vi "test-filter.vi"() -> ()   [LabVIEW 2019]
uses:
  <vilib>/Rock Robotics/WPI/ThirdParty/JAS_Junk/TrajLib/LINEAR_FILTER.ctl
  <vilib>/Rock Robotics/WPI/ThirdParty/JAS_Junk/TrajLib/Trajectory_Library.lvlib
panel:
  in  "Random noise amplitude":bool
  out "time diff":u32
  out "High BW2":T1 {"Outputs" format="%13.5p"; "Inputs" format="%13.5p"; "OutputGains" format="%13.5p"; "InputGains" format="%13.5p"}
  in  "noise Offset - millliseconds":dbl format="%14.5g"
  out "Cutoff Freq":dbl format="%14.5g"
  out "High BW1":T1 {"Outputs" format="%13.5p"; "Inputs" format="%13.5p"; "OutputGains" format="%13.5p"; "InputGains" format="%13.5p"}
  out "High Pass":T1 {"Outputs" format="%13.5p"; "Inputs" format="%13.5p"; "OutputGains" format="%13.5p"; "InputGains" format="%13.5p"}
  out "mov Avg":T1 {"Outputs" format="%13.5p"; "Inputs" format="%13.5p"; "OutputGains" format="%13.5p"; "InputGains" format="%13.5p"}
  in  "MovAvgSamp":i32 format="%14.5g"
  out "BW 2":T1 {"Outputs" format="%13.5p"; "Inputs" format="%13.5p"; "OutputGains" format="%13.5p"; "InputGains" format="%13.5p"}
  out "BW 1":T1 {"Outputs" format="%13.5p"; "Inputs" format="%13.5p"; "OutputGains" format="%13.5p"; "InputGains" format="%13.5p"}
  out "Single pole":T1 {"Outputs" format="%13.5p"; "Inputs" format="%13.5p"; "OutputGains" format="%13.5p"; "InputGains" format="%13.5p"}
  in  "Noise Amplitude":dbl(slide)=1.0 scale=0.0..10.0
  in  "TimeConstant":dbl format="%14.5g"
  in  "Noise Frequency":dbl(slide)=0.2 min=0.1 max=1000.0 step=0.5 scale=0.1..1000.0 scale format="%14.5g"
  out "Waveform Chart":T2(graph)
  in  "Primary Frequency":dbl(slide)=0.2 min=0.1 max=1000.0 step=0.5 scale=0.1..10.0 scale format="%14.5g"
  in  "Amplitude":dbl(slide)=1.0 scale=0.0..10.0
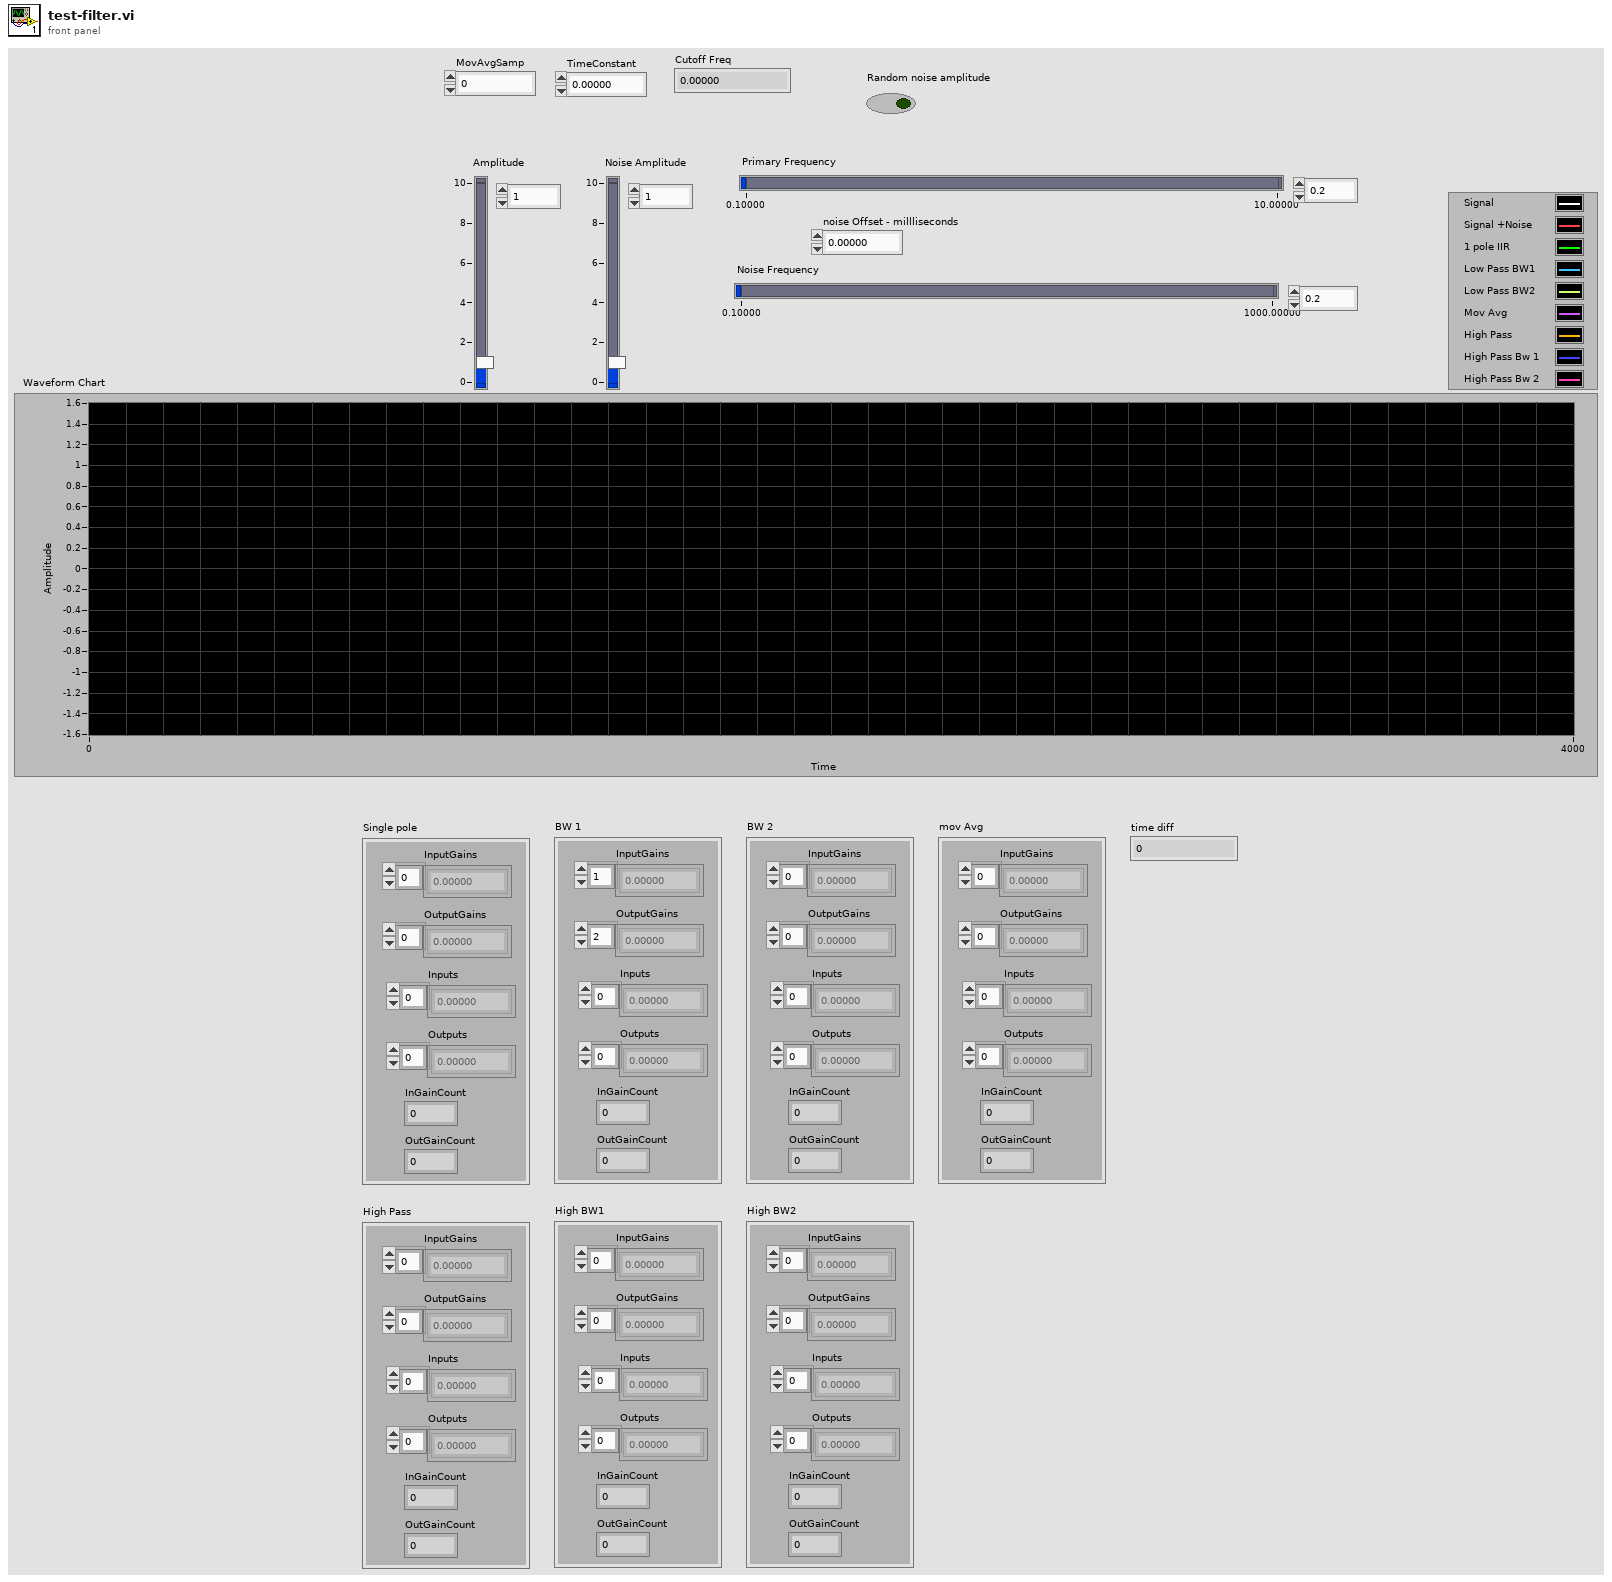
[diagram p1: front panel]
types:
  T1 = typedef "Trajectory_Library.lvlib/LINEAR_FILTER.ctl" = cluster{"InputGains":dbl[], "OutputGains":dbl[], "Inputs":dbl[], "Outputs":dbl[], "InGainCount":i32, "OutGainCount":i32}
  T2 = cluster{dbl, dbl, "Output":dbl, "Output":dbl, "Output":dbl, "Output":dbl, "Output":dbl, "Output":dbl, "Output":dbl}
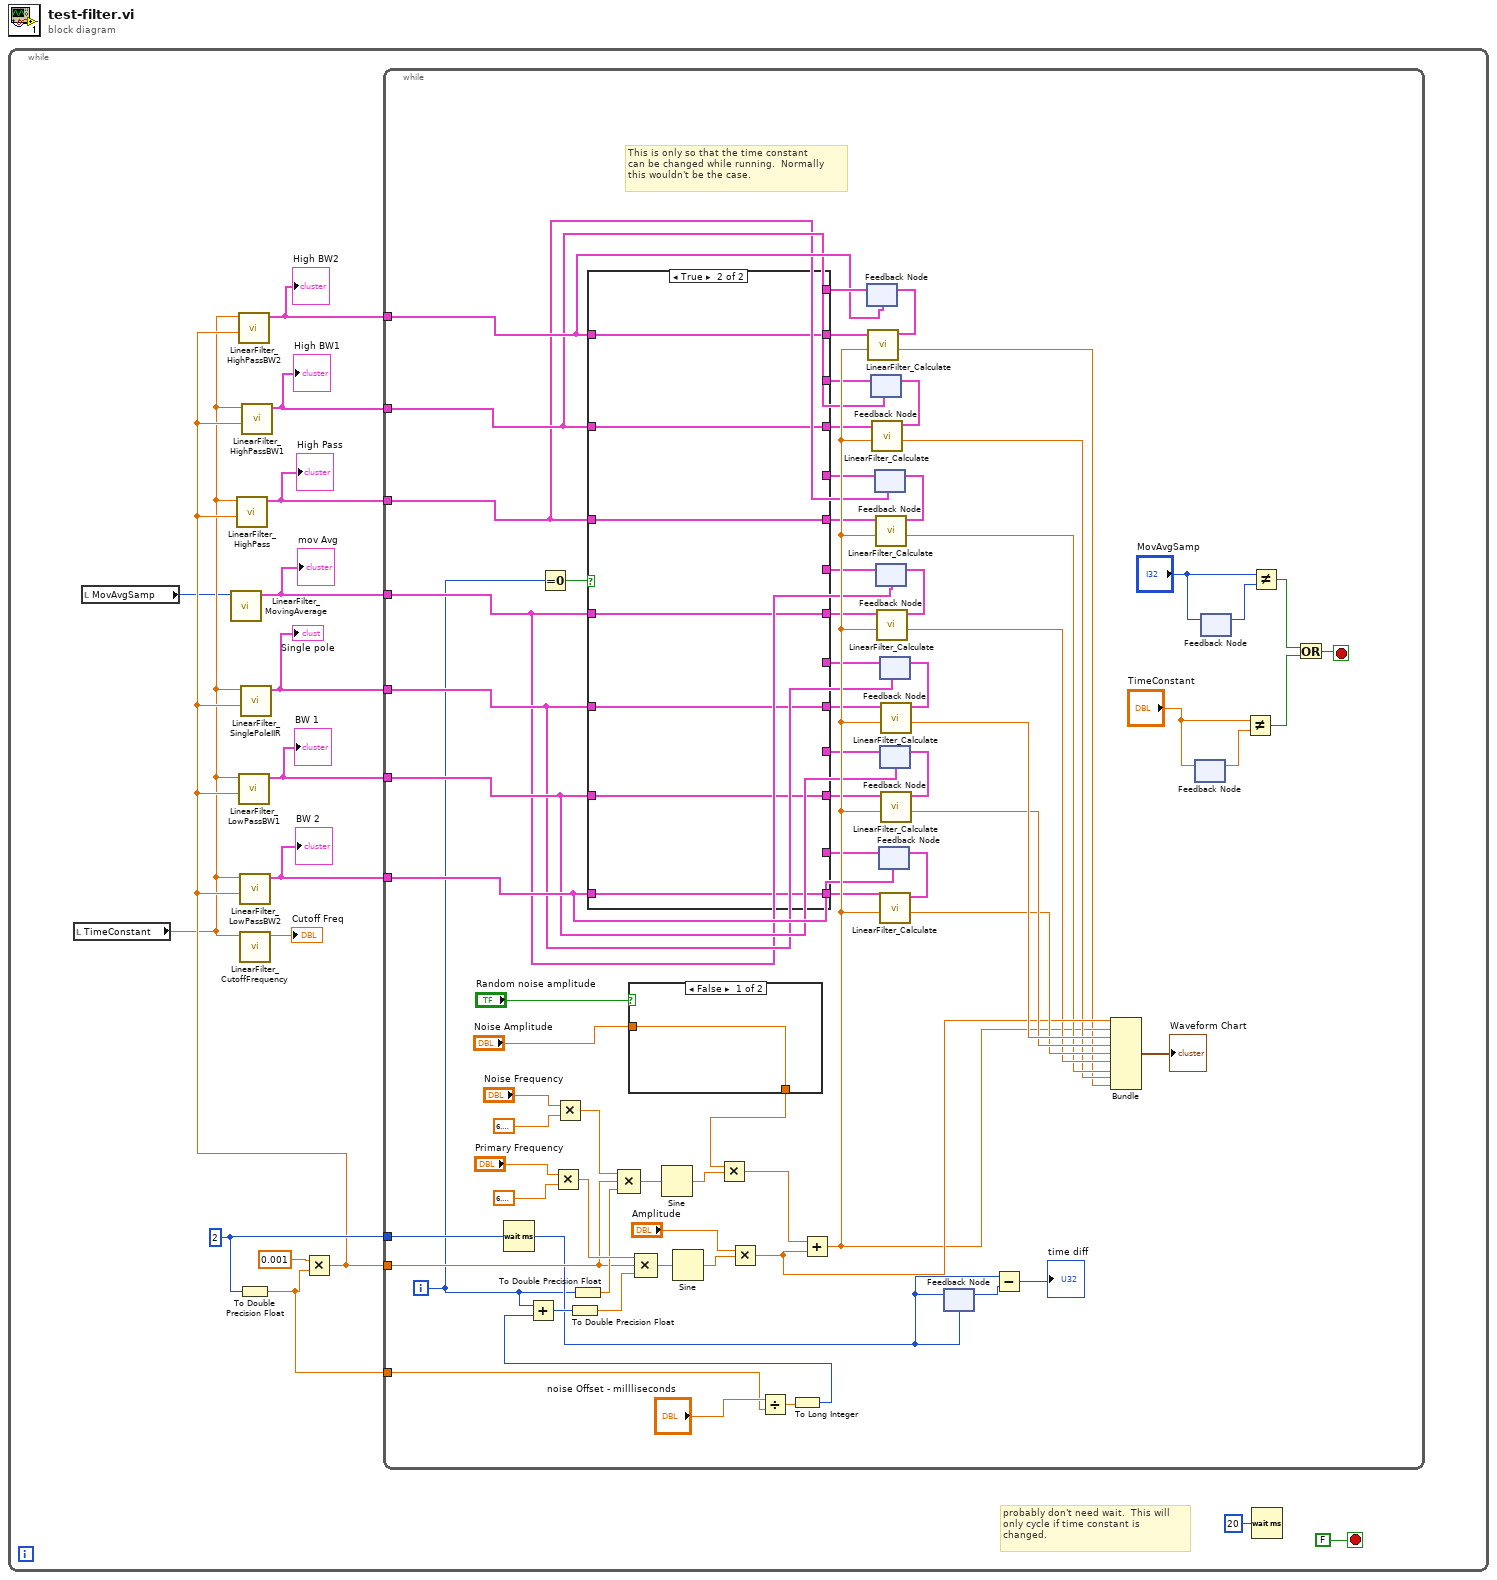
[diagram p0: block diagram]
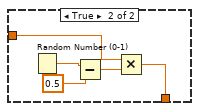
[diagram p2: hidden frame]
diagram:
  n1 = while {
    stop <- FALSE stop-if-true
    w15 = u32 2 ("milliseconds to wait")
    # "probably don't need wait.  This will \nonly cycle if time constant is\nchanged."
    n2 = local read "TimeConstant"() -> (w3:dbl)
    n3 = local read "MovAvgSamp"() -> (w2:i32)
    n4 = call <vilib>:"LinearFilter_MovingAverage.vi"("Samples"=w2) -> ("LINEAR_FILTER"=w12:T1)  [unwired: 10 in]
    "mov Avg" <- w12
    n5 = call <vilib>:"LinearFilter_CutoffFrequency.vi"("TimeConstant"=w3) -> ("Cutoff Freq"=→"Cutoff Freq":dbl)  [unwired: 10 in]
    n6 = To Double Precision Float(number=w15) -> (double precision float=w9:dbl)
    n7 = Multiply(x=0.001 ("value"), y=w9) -> (x*y=w8:dbl)
    n8 = call <vilib>:"LinearFilter_HighPass.vi"("SamplePeriod"=w8, "TimeConstant"=w3) -> ("LINEAR_FILTER"=w11:T1)  [unwired: 9 in]
    "High Pass" <- w11
    n9 = call <vilib>:"LinearFilter_HighPassBW2.vi"("SamplePeriod"=w8, "TimeConstant"=w3) -> ("LINEAR_FILTER"=w7:T1)  [unwired: 9 in]
    "High BW2" <- w7
    n10 = call <vilib>:"LinearFilter_LowPassBW1.vi"("SamplePeriod"=w8, "TimeConstant"=w3) -> ("LINEAR_FILTER"=w14:T1)  [unwired: 9 in]
    "BW 1" <- w14
    n11 = call <vilib>:"LinearFilter_LowPassBW2.vi"("SamplePeriod"=w8, "TimeConstant"=w3) -> ("LINEAR_FILTER"=w13:T1)  [unwired: 9 in]
    "BW 2" <- w13
    n12 = call <vilib>:"LinearFilter_SinglePoleIIR.vi"("SamplePeriod"=w8, "TimeConstant"=w3) -> ("LINEAR_FILTER"=w1:T1)  [unwired: 8 in, 1 out]
    "Single pole" <- w1
    n13 = call <vilib>:"LinearFilter_HighPassBW1.vi"("SamplePeriod"=w8, "TimeConstant"=w3) -> ("LINEAR_FILTER"=w10:T1)  [unwired: 9 in]
    "High BW1" <- w10
    n14 = while {
      tunnel: w15 -> [w84]
      tunnel: w8 -> [w76]
      tunnel: w14 -> [w27]
      tunnel: w13 -> [w28]
      tunnel: w12 -> [w25]
      tunnel: w11 -> [w22]
      tunnel: w10 -> [w23]
      tunnel: w9 -> [w57]
      tunnel: w7 -> [w24]
      tunnel: w1 -> [w26]
      i -> [w20]
      stop <- w45 stop-if-true
      # "This is only so that the time constant\ncan be changed while running.  Normally\nthis wouldn't be the case."
      n15 = Wait (ms)(milliseconds to wait=w84) -> (millisecond timer value=w51:u32)
      n16 = Equal To 0?(x=w20) -> (x = 0?=w21:bool)
      n17 = Multiply(x="Primary Frequency", y=6.283185307179586) -> (x*y=w78:dbl)
      n18 = Multiply(x="Noise Frequency", y=6.283185307179586) -> (x*y=w79:dbl)
      n19 = To Double Precision Float(number=w20) -> (double precision float=w77:dbl)
      n20 = Compound Arithmetic op=MULTIPLY(w79, w76, w77) -> (w81:dbl)
      n21 = case shown="False" "Random noise amplitude" {
        tunnel: "Noise Amplitude" -> [w91 w93]
        tunnel: [w91 w92] -> w17
        frame False {
        }
        frame True {
          n22 = Random Number (0-1)() -> (number: 0 to 1=w96:dbl)
          n23 = Subtract(x=w96, y=0.5) -> (x-y=w94:dbl)
          n24 = Multiply(x=w93, y=w94) -> (x*y=w92:dbl)
        }
      }
      n25 = Sine(x=w81) -> (sin(x)=w80:dbl)
      n26 = Multiply(x=w17, y=w80) -> (x*y=w75:dbl)
      n27 = Divide(x="noise Offset - millliseconds", y=w57) -> (x/y=w59:dbl)
      n28 = To Long Integer(number=w59) -> (32bit integer=w56:i32)
      n29 = Add(x=w20, y=w56) -> (x+y=w61:i32)
      n30 = To Double Precision Float(number=w61) -> (double precision float=w60:dbl)
      n31 = Compound Arithmetic op=MULTIPLY(w78, w76, w60) -> (w90:dbl)
      n32 = Sine(x=w90) -> (sin(x)=w89:dbl)
      n33 = Multiply(x="Amplitude", y=w89) -> (x*y=w68:dbl)
      n34 = Add(x=w75, y=w68) -> (x+y=w54:dbl)
      n35 = feedback #1(w24) -> (w41:T1)
      n36 = feedback #2(w23) -> (w39:T1)
      n37 = feedback #3(w22) -> (w37:T1)
      n38 = feedback #4(w25) -> (w35:T1)
      n39 = feedback #5(w28) -> (w29:T1)
      n40 = feedback #6(w26) -> (w33:T1)
      n41 = feedback #7(w27) -> (w31:T1)
      n42 = case shown="True" w21 {
        tunnel: [w103 w110] -> w42
        tunnel: w41 -> [w103 _]
        tunnel: [w102 w109] -> w40
        tunnel: w39 -> [w102 _]
        tunnel: [w101 w108] -> w38
        tunnel: w37 -> [w101 _]
        tunnel: [w100 w107] -> w36
        tunnel: w35 -> [w100 _]
        tunnel: [w99 w106] -> w34
        tunnel: w33 -> [w99 _]
        tunnel: [w98 w105] -> w32
        tunnel: w31 -> [w98 _]
        tunnel: [w97 w104] -> w30
        tunnel: w29 -> [w97 _]
        tunnel: w24 -> [_ w110]
        tunnel: w23 -> [_ w109]
        tunnel: w22 -> [_ w108]
        tunnel: w25 -> [_ w107]
        tunnel: w26 -> [_ w106]
        tunnel: w27 -> [_ w105]
        tunnel: w28 -> [_ w104]
        frame False {
        }
        frame True {
        }
      }
      n43 = call <vilib>:"LinearFilter_Calculate.vi"("Input"=w54, "In LINEAR_FILTER"=w42) -> ("Output"=w53:dbl, "Out LINEAR_FILTER"=w55:T1)  [unwired: 8 in]
      n44 = feedback-in #1(w55) -> ()
      n45 = call <vilib>:"LinearFilter_Calculate.vi"("Input"=w54, "In LINEAR_FILTER"=w40) -> ("Output"=w62:dbl, "Out LINEAR_FILTER"=w63:T1)  [unwired: 8 in]
      n46 = feedback-in #2(w63) -> ()
      n47 = call <vilib>:"LinearFilter_Calculate.vi"("Input"=w54, "In LINEAR_FILTER"=w38) -> ("Output"=w64:dbl, "Out LINEAR_FILTER"=w65:T1)  [unwired: 8 in]
      n48 = feedback-in #3(w65) -> ()
      n49 = call <vilib>:"LinearFilter_Calculate.vi"("Input"=w54, "In LINEAR_FILTER"=w36) -> ("Output"=w66:dbl, "Out LINEAR_FILTER"=w67:T1)  [unwired: 8 in]
      n50 = feedback-in #4(w67) -> ()
      n51 = call <vilib>:"LinearFilter_Calculate.vi"("Input"=w54, "In LINEAR_FILTER"=w30) -> ("Output"=w72:dbl, "Out LINEAR_FILTER"=w69:T1)  [unwired: 8 in]
      n52 = feedback-in #5(w69) -> ()
      n53 = call <vilib>:"LinearFilter_Calculate.vi"("Input"=w54, "In LINEAR_FILTER"=w34) -> ("Output"=w74:dbl, "Out LINEAR_FILTER"=w71:T1)  [unwired: 8 in]
      n54 = feedback-in #6(w71) -> ()
      n55 = call <vilib>:"LinearFilter_Calculate.vi"("Input"=w54, "In LINEAR_FILTER"=w32) -> ("Output"=w73:dbl, "Out LINEAR_FILTER"=w70:T1)  [unwired: 8 in]
      n56 = feedback-in #7(w70) -> ()
      n57 = feedback-in #8(w51) -> ()
      n58 = feedback #8(w51) -> (w52:u32)
      n59 = Subtract(x=w51, y=w52) -> (x-y=→"time diff":u32)
      n60 = Bundle(w68, w54, "Output"=w74, "Output"=w73, "Output"=w72, "Output"=w66, "Output"=w64, "Output"=w62, "Output"=w53) -> (→"Waveform Chart":T2)  [unwired: 1 in]
      n61 = feedback-in #9("TimeConstant") -> ()
      n62 = feedback #9() -> (w48:dbl)  [unwired: 1 in]
      n63 = feedback #10() -> (w47:i32)  [unwired: 1 in]
      n64 = feedback-in #10("MovAvgSamp") -> ()
      n65 = Not Equal?(x="TimeConstant", y=w48) -> (x != y?=w43:bool)
      n66 = Not Equal?(x="MovAvgSamp", y=w47) -> (x != y?=w44:bool)
      n67 = Or(x=w44, y=w43) -> (x .or. y?=w45:bool)
    }
    n68 = Wait (ms)(milliseconds to wait=u32 20) -> ()  [unwired: 1 out]
  }
